vi "Message to String.vi"(8 "error in":errorcluster, 11 "message in":T1) -> (0 "error out":errorcluster, 3 "string out":string)   [LabVIEW 2017, in "Lock-In Amplifier Example Shared.lvlib"]
uses:
  Lock-In Amplifier Example Shared.lvlib
  message.ctl
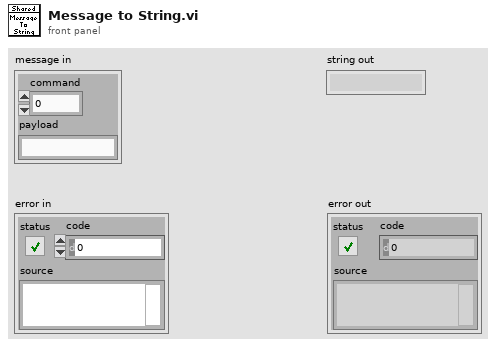
[diagram p1: front panel]
types:
  T1 = typedef "Lock-In Amplifier Example Shared.lvlib/message.ctl" = cluster{"command":u32, "payload":string}
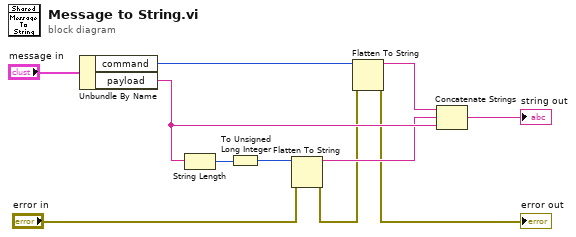
[diagram p0: block diagram]
diagram:
  n1 = Unbundle By Name("message in") -> ("command"=w8:u32, "payload"=w6:string)
  n2 = String Length(string=w6) -> (length=w10:i32)
  n3 = To Unsigned Long Integer(number=w10) -> (unsigned 32bit integer=w9:u32)
  n4 = Flatten To String(anything=w9, error in (no error)="error in") -> (data string=w5:string, error out=w3:errorcluster)  [unwired: 2 in, 1 out]
  n5 = Flatten To String(anything=w8, error in (no error)=w3) -> (data string=w7:string, error out=→"error out":errorcluster)  [unwired: 2 in, 1 out]
  n6 = Concatenate Strings(w7, w5, w6) -> (→"string out":string)
